vi "Send_Trajectory.vi"(8 "error in (no error)":errorcluster, 9 "Advanced":bool, 10 "TrajectoryPoint":T1) -> (0 "error out":errorcluster)   [LabVIEW 2019]
uses:
  <vilib>/Utility/error.llb/Error Cluster From Error Code.vi
  <vilib>/ErrorRing/Error Ring.xnode
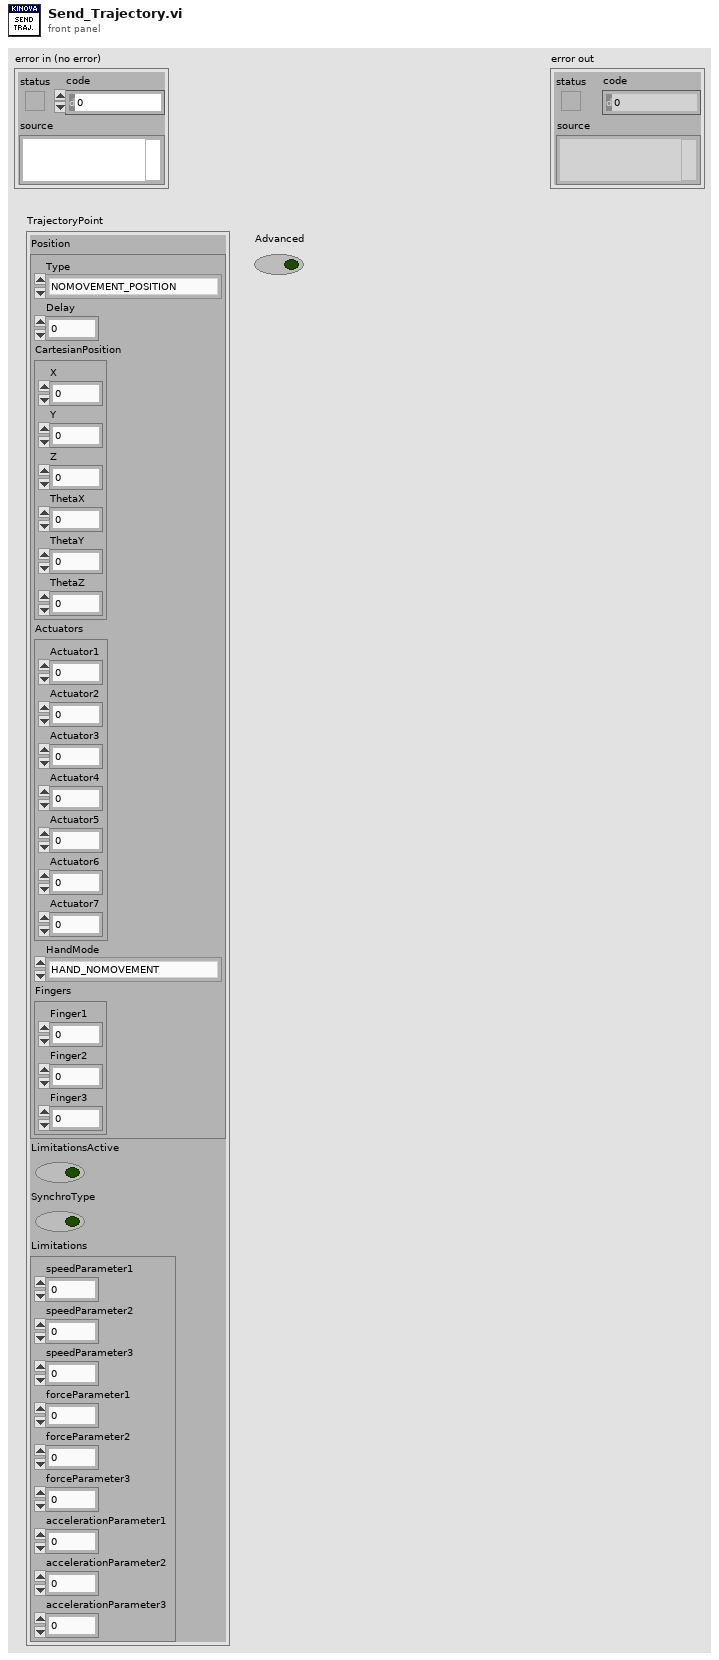
[diagram p1: front panel]
types:
  T1 = cluster{"Position":cluster{"Type":enum16{"NOMOVEMENT_POSITION", "CARTESIAN_POSITION", "ANGULAR_POSITION", "RETRACTED", "PREDEFINED1", "PREDEFINED2", "PREDEFINED3", "CARTESIAN_VELOCITY", "ANGULAR_VELOCITY", "PREDEFINED4", "PREDEFINED5", "ANY_TRAJECTORY", "TIME_DELAY"}, "Delay":sgl, "CartesianPosition":cluster{"X":sgl, "Y":sgl, "Z":sgl, "ThetaX":sgl, "ThetaY":sgl, "ThetaZ":sgl}, "Actuators":cluster{"Actuator1":sgl, "Actuator2":sgl, "Actuator3":sgl, "Actuator4":sgl, "Actuator5":sgl, "Actuator6":sgl, "Actuator7":sgl}, "HandMode":enum16{"HAND_NOMOVEMENT", "POSITION_MODE", "VELOCITY_MODE", "NO_FINGER", "ONE_FINGER", "TWO_FINGERS", "THREE_FINGERS"}, "Fingers":cluster{"Finger1":sgl, "Finger2":sgl, "Finger3":sgl}}, "LimitationsActive":bool, "SynchroType":bool, "Limitations":cluster{"speedParameter1":sgl, "speedParameter2":sgl, "speedParameter3":sgl, "forceParameter1":sgl, "forceParameter2":sgl, "forceParameter3":sgl, "accelerationParameter1":sgl, "accelerationParameter2":sgl, "accelerationParameter3":sgl}}
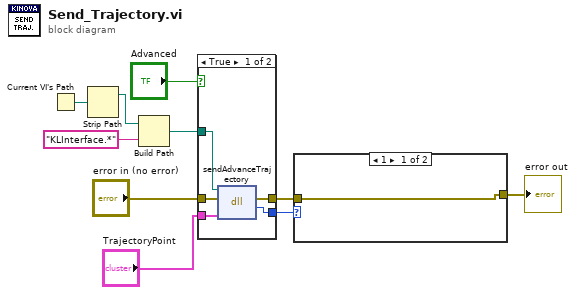
[diagram p0: block diagram]
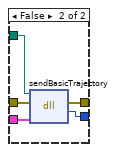
[diagram p2: hidden frame]
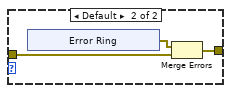
[diagram p3: hidden frame]
diagram:
  n1 = Current VI's Path() -> (path=w8:path)
  n2 = Strip Path(path=w8) -> (stripped path=w7:path)  [unwired: 1 out]
  n3 = Build Path(base path=w7, name or relative path="KLInterface.*") -> (appended path=w2:path)
  n4 = case shown="True" "Advanced" {
    tunnel: "error in (no error)" -> [w15 w20]
    tunnel: [w14 w19] -> w6
    tunnel: [w13 w18] -> w5
    tunnel: "TrajectoryPoint" -> [w12 w17]
    tunnel: w2 -> [w11 w16]
    frame True {
      n5 = dll-call lib="C:/Users/mcjssdcc/source/repos/Kinova Labview Interface/Debug/KLInterface.dll" fn="sendAdvanceTrajectory"(path in=w11, error in=w15, "point"=w12) -> (error out=w14:errorcluster, "return type"=w13:i32)  [unwired: 2 in, 1 out]
    }
    frame False {
      n6 = dll-call lib="C:/Users/mcjssdcc/source/repos/Kinova Labview Interface/Debug/KLInterface.dll" fn="sendBasicTrajectory"(path in=w16, error in=w20, "point"=w17) -> (error out=w19:errorcluster, "return type"=w18:i32)  [unwired: 2 in, 1 out]
    }
  }
  n7 = case shown="1" w5 {
    tunnel: [w21 w23] -> w4
    tunnel: w6 -> [w21 w22]
    frame 1 {
    }
    frame Default {
      n8 = xnode "Error Ring"() -> ("error out"=w24:errorcluster)
      n9 = Merge Errors(w24, w22) -> (w23:errorcluster)
    }
  }
  "error out" <- w4
